vi "Xsens Quaternion (SubVI).vi"(5 "DATA in (Hex)":string) -> (0 "Channel Units":string[](array[string])=["NA", "YYYY", "MM", "dd", "hh", "mm", "ss", "NA", "ns", "NA", "NA", "NA", "NA", "DD", "DD", "mm", "mm", "mm", "mm"], 1 "Channel DataTypes":string[](array[string])=["NA", "YYYY", "MM", "dd", "hh", "mm", "ss", "NA", "ns", "NA", "NA", "NA", "NA", "DD", "DD", "mm", "mm", "mm", "mm"], 2 "Quaternion":string[](array[string]), 3 "Channel Names":string[](array[string]))   [LabVIEW 2019]
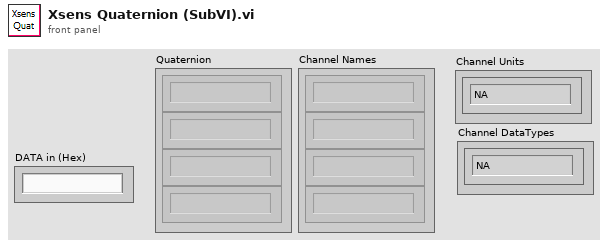
[diagram p1: front panel]
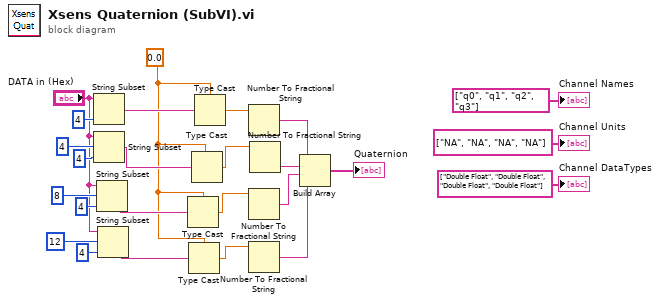
[diagram p0: block diagram]
diagram:
  w13 = sgl 0.0
  n1 = String Subset(string="DATA in (Hex)", length (rest)=4 ("length (rest)")) -> (substring=w24:string)  [unwired: 1 in]
  n2 = String Subset(string="DATA in (Hex)", offset (0)=4, length (rest)=4 ("length (rest)")) -> (substring=w19:string)
  n3 = String Subset(string="DATA in (Hex)", offset (0)=8, length (rest)=4 ("length (rest)")) -> (substring=w18:string)
  n4 = String Subset(string="DATA in (Hex)", offset (0)=12, length (rest)=4 ("length (rest)")) -> (substring=w15:string)
  n5 = Type Cast(type=w13, x=w18) -> (*(type *) &x=w8:sgl)
  n6 = Type Cast(type=w13, x=w15) -> (*(type *) &x=w6:sgl)
  n7 = Type Cast(type=w13, x=w19) -> (*(type *) &x=w10:sgl)
  n8 = Type Cast(type=w13, x=w24) -> (*(type *) &x=w12:sgl)
  n9 = Number To Fractional String(number=w12) -> (F-format string=w11:string)  [unwired: 3 in]
  n10 = Number To Fractional String(number=w8) -> (F-format string=w7:string)  [unwired: 3 in]
  n11 = Number To Fractional String(number=w6) -> (F-format string=w5:string)  [unwired: 3 in]
  n12 = Number To Fractional String(number=w10) -> (F-format string=w9:string)  [unwired: 3 in]
  n13 = Build Array(w11, w9, w7, w5) -> (→"Quaternion":string[])
  "Channel Names" <- string[] ["q0", "q1", "q2", "q3"] ("Channel Names")
  "Channel Units" <- string[] ["NA", "NA", "NA", "NA"] ("Channel Names")
  "Channel DataTypes" <- string[] ["Double Float", "Double Float", "Double Float", "Double Float"] ("Channel Names")
